vi "ActiveObjects_DynamicEvents_ControlWindow_6x8x6_Singleton.vi"(1 "ShowProcessWindow":bool, 5 "error in (no error)":errorcluster) -> (19 "error out":errorcluster)   [LabVIEW 2010]
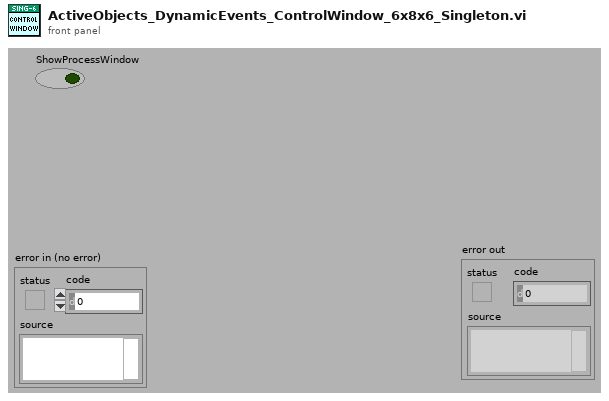
[diagram p1: front panel]
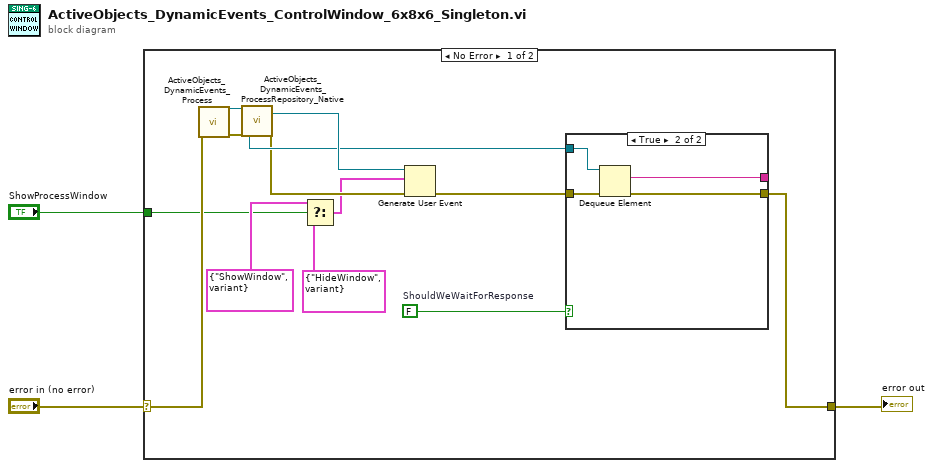
[diagram p0: block diagram]
diagram:
  n1 = case shown="No Error" "error in (no error)" {
    selector: "error in (no error)" -> [w9 w22]
    tunnel: [w8 w22] -> w2
    tunnel: "ShowProcessWindow" -> [w5 _]
    frame No Error {
      w15 = FALSE  # ShouldWeWaitForResponse
      n2 = call "ActiveObjects_DynamicEvents_Process.vi"("error in (no error)"=w9) -> ("reference out"=w11:refnum<class>, "error out"=w10:errorcluster)  [unwired: 17 in]
      n3 = call "ActiveObjects_DynamicEvents_ProcessRepository_Native.vi"("reference in"=w11, "error in (no error)"=w10) -> ("QueueFromProcess"=w13:refnum<queue>, "EventsToProcess"=w16:refnum<user-event>, "error out"=w12:errorcluster)  [unwired: 10 in, 5 out]
      n4 = Select(t=cluster{"Command":string, "Data":variant} {"Command"="ShowWindow", "Data"=variant} ("MessageToProcess"), s=w5, f=cluster{"Command":string, "Data":variant} {"Command"="HideWindow", "Data"=variant} ("MessageToProcess")) -> (s? t:f=w4:cluster{"Command":string, "Data":variant})
      n5 = Generate User Event(user event=w16, event data cluster=w4, error in=w12) -> (error out=w14:errorcluster)  [unwired: 1 out]
      n6 = case shown="True" w15 {
        tunnel: w14 -> [w17 w21]
        tunnel: w13 -> [_ w20]
        tunnel: [_ w19] -> _
        tunnel: [w17 w18] -> w8
        frame False {
        }
        frame True {
          n7 = Dequeue Element(queue=w20, error in (no error)=w21) -> (element=w19:string, error out=w18:errorcluster)  [unwired: 1 in, 2 out]
        }
      }
    }
    frame Error {
    }
  }
  "error out" <- w2
